vi "SRX_Config_ALL.vi"(11 "Talon Setup":T1={"Open Data"={"SRX ID"=0, "Invert Output"=FALSE}, "Current Config Data"={"Enable Current Limit?"=FALSE, "Peak Current (Amps)"=0, "Peak Current Maximum Duration (ms)"=0, "Continuous Current Limit (Amps)"=0}, "Sensor Config"={"Feedback Device"=1, "PhaseSensor"=FALSE}, "Hard Limits"={"Fwd Enable"=FALSE, "Rev Enable"=FALSE, "Fwd NO-NC"=enum."Normally Open", "Rev NO-NC"=enum."Normally Open"}, "Motion Magic Config Data"={"Cruise Velocity"=0, "Acceleration"=0}, "PIDF"={"P"=0.0, "I"=0.0, "D"=0.0, "F"=0.0, "I Zone"=0.0}, "Maximum Integral Accumulator Value"=0.0, "AllowableClosedLoop"=0, "Limits"={"Max"=0, "Min"=0, "Max Enable"=FALSE, "Min Enable"=FALSE}, "Output Config"={"Invert?"=FALSE, "Neutral Mode"=enum."EEPROMSetting", "Deadband (-1to1)"=0.0, "Ramp Time Off to Full (S)"=0.0, "Peak  (-1to1)"={"Forward"=1.0, "Reverse"=-1.0}, "Nominal  (-1to1)"={"Forward"=0.0, "Reverse"=0.0}}} {"Sensor Config"."Feedback Device" items=["None"=-1, "QuadEncoder"=0, "Analog"=2, "Tachometer"=4, "Pulse Width Encoded Position"=8, "Sensor Sum (S0 + S1)"=9, "Sensor Difference (D0 - D1)"=10, "Remote Source 0"=11, "Remote Source 1"=12, "Software Emulated"=15]}) -> (3 "PhoenixMotorControlDevRef Out":T14)   [LabVIEW 2017]
uses:
  <vilib>/Rock Robotics/WPI/MotorControl/WPI_MotorControlDeviceRef.ctl
  <vilib>/Rock Robotics/WPI/MotorControl/WPI_MotorControlType.ctl
  <vilib>/Rock Robotics/SystemInterfaces/DIO/FPGA_DIOPWMChannel.ctl
  <vilib>/Rock Robotics/WPI/PWM/WPI_PWMDeadband.ctl
  <vilib>/Rock Robotics/SystemInterfaces/DIO/FPGA_DIOChannel.ctl
  Competition Code/RoboRio Code/TypeDef/CLUSTER_Talon_Setup.ctl
  TypeDefs SRX/Cluster_SRX_OPEN Data.ctl
  TypeDefs SRX/Cluster_SRX_Current Config.ctl
  TypeDefs SRX/Cluster_SRX_Sensor Config.ctl
  System Drivers/Phoenix-LabVIEW/Motor Controller/Controls/CTRE_Phoenix_MotorControl_FeedbackDevice.ctl
  TypeDefs SRX/Cluster_SRX_Config Hard Limits.ctl
  System Drivers/Phoenix-LabVIEW/Motor Controller/Controls/CTRE_Phoenix_MotorControl_LimitSwitchNormal.ctl
  TypeDefs SRX/Cluster_SRX_Motion Magic Config Data.ctl
  TypeDefs SRX/Cluster_SRX_PIDF.ctl
  TypeDefs SRX/Cluster_SRX_Config Soft Limits.ctl
  TypeDefs SRX/Cluster_SRX_Config Voltage Output.ctl
  System Drivers/Phoenix-LabVIEW/Motor Controller/Controls/CTRE_Phoenix_MotorControl_NeutralMode.ctl
  TypeDefs SRX/Cluster_SRX_Forward and Reverse.ctl
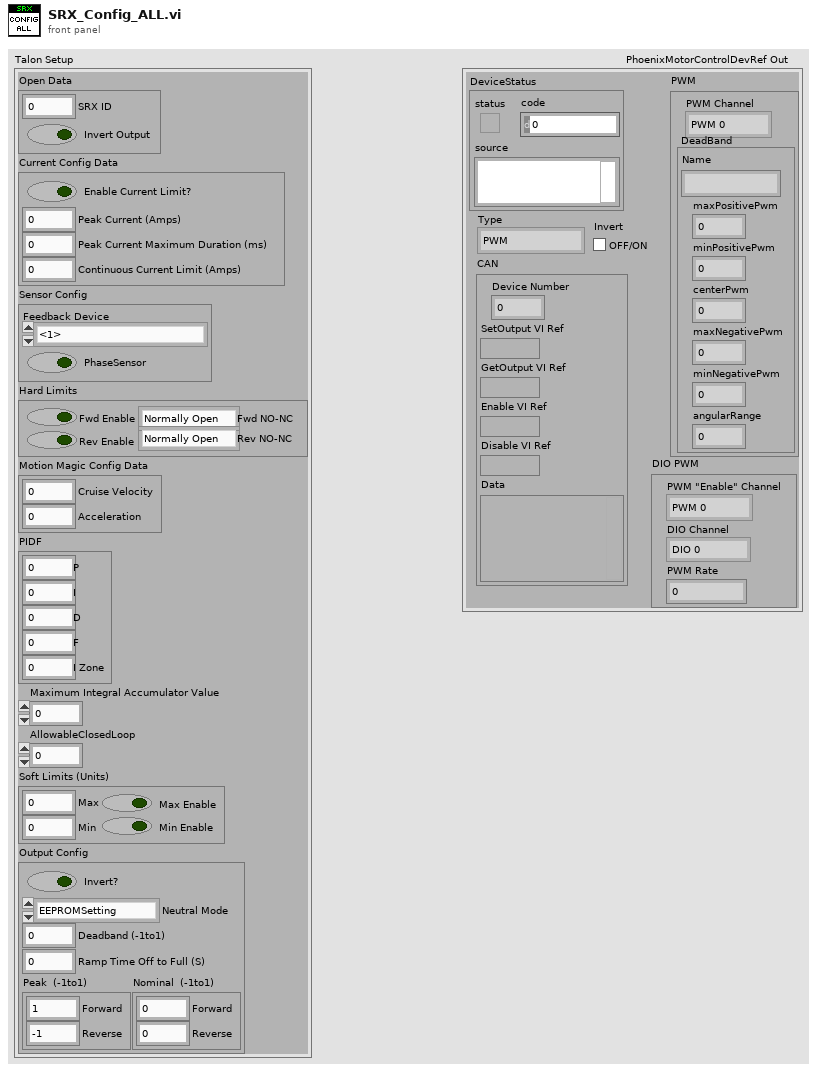
[diagram p1: front panel]
types:
  T1 = typedef "CLUSTER_Talon_Setup.ctl" = cluster{"Open Data":T2, "Current Config Data":T3, "Sensor Config":T4, "Hard Limits":T6, "Motion Magic Config Data":T8, "PIDF":T9, "Maximum Integral Accumulator Value":dbl, "AllowableClosedLoop":i32, "Limits":T10, "Output Config":T11}
  T2 = typedef "Cluster_SRX_OPEN Data.ctl" = cluster{"SRX ID":u8, "Invert Output":bool}
  T3 = typedef "Cluster_SRX_Current Config.ctl" = cluster{"Enable Current Limit?":bool, "Peak Current (Amps)":i32, "Peak Current Maximum Duration (ms)":i32, "Continuous Current Limit (Amps)":i32}
  T4 = typedef "Cluster_SRX_Sensor Config.ctl" = cluster{"Feedback Device":T5, "PhaseSensor":bool}
  T5 = typedef "CTRE_Phoenix_MotorControl_FeedbackDevice.ctl" = i8
  T6 = typedef "Cluster_SRX_Config Hard Limits.ctl" = cluster{"Fwd Enable":bool, "Rev Enable":bool, "Fwd NO-NC":T7, "Rev NO-NC":T7}
  T7 = typedef "CTRE_Phoenix_MotorControl_LimitSwitchNormal.ctl" = enum16{"Normally Open", "Normally Closed", "Disabled"}
  T8 = typedef "Cluster_SRX_Motion Magic Config Data.ctl" = cluster{"Cruise Velocity":i32, "Acceleration":i32}
  T9 = typedef "Cluster_SRX_PIDF.ctl" = cluster{"P":dbl, "I":dbl, "D":dbl, "F":dbl, "I Zone":dbl}
  T10 = typedef "Cluster_SRX_Config Soft Limits.ctl" = cluster{"Max":i32, "Min":i32, "Max Enable":bool, "Min Enable":bool}
  T11 = typedef "Cluster_SRX_Config Voltage Output.ctl" = cluster{"Invert?":bool, "Neutral Mode":T12, "Deadband (-1to1)":dbl, "Ramp Time Off to Full (S)":dbl, "Peak  (-1to1)":T13, "Nominal  (-1to1)":T13}
  T12 = typedef "CTRE_Phoenix_MotorControl_NeutralMode.ctl" = enum8{"EEPROMSetting", "Override to Coast", "Override to Brake"}
  T13 = typedef "Cluster_SRX_Forward and Reverse.ctl" = cluster{"Forward":dbl, "Reverse":dbl}
  T14 = typedef "WPI_MotorControlDeviceRef.ctl" = cluster{"DeviceStatus":errorcluster, "Type":T15, "PWM":cluster{"PWM Channel":T16, "DeadBand":T17}, "CAN":cluster{"Device Number":u8, "SetOutput VI Ref":variant, "GetOutput VI Ref":variant, "Enable VI Ref":variant, "Disable VI Ref":variant, "Data":variant}, "Invert":bool, "DIO PWM":cluster{"PWM \"Enable\" Channel":T16, "DIOChannel":T18, "PWM Rate":dbl}}
  T15 = typedef "WPI_MotorControlType.ctl" = enum16{"PWM", "CAN", "DIO PWM"}
  T16 = typedef "FPGA_DIOPWMChannel.ctl" = enum8{"PWM 0", "PWM 1", "PWM 2", "PWM 3", "PWM 4", "PWM 5", "PWM 6", "PWM 7", "PWM 8", "PWM 9", "PWM MXP 0", "PWM MXP 1", "PWM MXP 2", "PWM MXP 3", "PWM MXP 4", "PWM MXP 5", "PWM MXP 6", "PWM MXP 7", "PWM MXP 8", "PWM MXP 9", "Invalid"}
  T17 = typedef "WPI_PWMDeadband.ctl" = cluster{"Name":string, "maxPositivePwm":i32, "minPositivePwm":i32, "centerPwm":i32, "maxNegativePwm":i32, "minNegativePwm":i32, "angularRange":u16}
  T18 = typedef "FPGA_DIOChannel.ctl" = enum8{"DIO 0", "DIO 1", "DIO 2", "DIO 3", "DIO 4", "DIO 5", "DIO 6", "DIO 7", "DIO 8", "DIO 9", "DIO MXP 0", "DIO MXP 1", "DIO MXP 2", "DIO MXP 3", "DIO MXP 4", "DIO MXP 5", "DIO MXP 6", "DIO MXP 7", "DIO MXP 8", "DIO MXP 9", "DIO MXP 10", "DIO MXP 11", "DIO MXP 12", "DIO MXP 13", "DIO MXP 14", "DIO MXP 15", "SPI Port CS1", "SPI Port CS2", "SPI Port CS3", "SPI Port MISO", "SPI Port MOSI", "Invalid"}
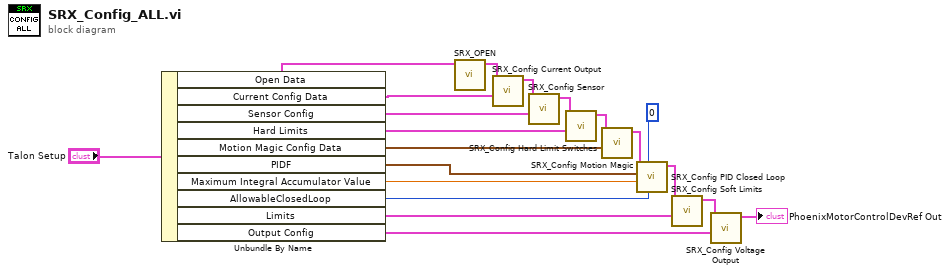
[diagram p0: block diagram]
diagram:
  n1 = Unbundle By Name("Talon Setup") -> ("Open Data"=w19:T2, "Current Config Data"=w10:T3, "Sensor Config"=w9:T4, "Hard Limits"=w8:T6, "Motion Magic Config Data"=w7:T8, "PIDF"=w6:T9, "Maximum Integral Accumulator Value"=w5:dbl, "AllowableClosedLoop"=w1:i32, "Limits"=w4:T10, "Output Config"=w3:T11)
  n2 = call "SRX_OPEN.vi"("Open Data"=w19) -> ("PhoenixMotorControlDevRef Out"=w18:T14)  [unwired: 9 in, 1 out]
  n3 = call "SRX_Config Current Output.vi"("Current Config Data"=w10, "PhoenixMotorControlDevRef"=w18) -> ("PhoenixMotorControlDevRef Out"=w17:T14)  [unwired: 8 in, 1 out]
  n4 = call "SRX_Config Sensor.vi"("Sensor Config"=w9, "PhoenixMotorControlDevRef"=w17) -> ("PhoenixMotorControlDevRef Out"=w16:T14)  [unwired: 8 in, 1 out]
  n5 = call "SRX_Config Hard Limit Switches.vi"("Hard Limits"=w8, "PhoenixMotorControlDevRef"=w16) -> ("PhoenixMotorControlDevRef Out"=w15:T14)  [unwired: 8 in, 1 out]
  n6 = call "SRX_Config Motion Magic.vi"("Motion Magic Config Data"=w7, "PhoenixMotorControlDevRef"=w15) -> ("PhoenixMotorControlDevRef Out"=w14:T14)  [unwired: 8 in, 1 out]
  n7 = call "SRX_Config PID Closed Loop.vi"("AllowableClosedLoopError"=w1, "SlotIdx"=0, "Maximum Integral Accumulator Value"=w5, "PIDF"=w6, "PhoenixMotorControlDevRef"=w14) -> ("PhoenixMotorControlDevRef Out"=w13:T14)  [unwired: 5 in, 1 out]
  n8 = call "SRX_Config Soft Limits.vi"("Soft Limits (Units)"=w4, "PhoenixMotorControlDevRef"=w13) -> ("PhoenixMotorControlDevRef Out"=w12:T14)  [unwired: 8 in, 1 out]
  n9 = call "SRX_Config Voltage Output.vi"("Output Config"=w3, "PhoenixMotorControlDevRef"=w12) -> ("PhoenixMotorControlDevRef Out"=→"PhoenixMotorControlDevRef Out":T14)  [unwired: 8 in, 1 out]
